vi "Comments.Add Device Description.vi"(8 "error in (no error)":errorcluster, 11 "Control Experiment in":refnum<class "Control Experiment.lvclass">) -> (0 "error out":errorcluster, 3 "Control Experiment out":refnum<class "Control Experiment.lvclass">)   [LabVIEW 2016, in "Control Experiment.lvclass"]
uses:
  Control Experiment.lvclass
  Control Experiment.lvclass/Control Experiment.ctl
panel:
  out "Device Description":string
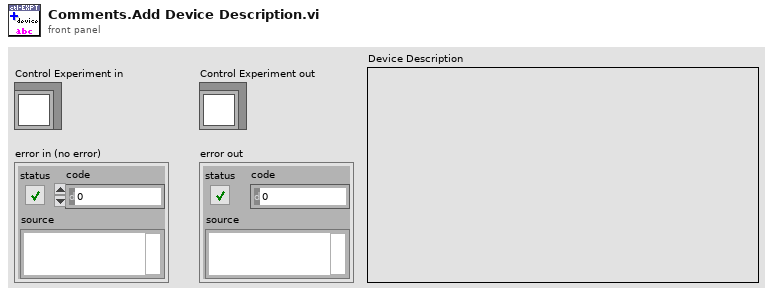
[diagram p1: front panel]
types:
  T1 = typedef "Control Experiment.lvclass/Instrument--enum.ctl" = enum16{"PPMS", "PPMS2", "MFP3D", "CYPHER", "THz1", "THz2", "MNK", "CF900", "JEOL", "AGILENT", "EBL"}
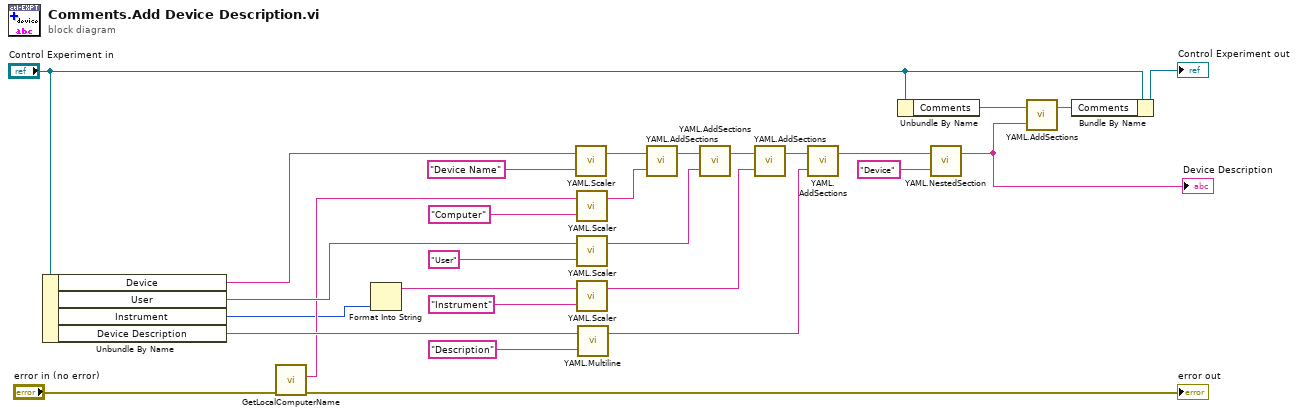
[diagram p0: block diagram]
diagram:
  n1 = Unbundle By Name("Control Experiment in") -> ("Device"=w8:string, "User"=w12:string, "Instrument"=w6:T1, "Device Description"=w17:string)
  n2 = call <userlib>:"GetLocalComputerName.vi"("error in (no error)"="error in (no error)") -> ("error out"=→"error out":errorcluster, "Name"=w10:string)  [unwired: 8 in, 1 out]
  n3 = Format Into String(w6) -> (resulting string=w15:string)  [unwired: 3 in, 1 out]
  n4 = call "YAML.Scaler.vi"("Key"="Device Name" ("string"), "Scaler"=w8) -> ("Output"=w26:string)  [unwired: 1 in]
  n5 = call "YAML.Scaler.vi"("Key"="Computer" ("string"), "Scaler"=w10) -> ("Output"=w18:string)  [unwired: 1 in]
  n6 = call "YAML.Scaler.vi"("Key"="User" ("string"), "Scaler"=w12) -> ("Output"=w20:string)  [unwired: 1 in]
  n7 = call "YAML.Scaler.vi"("Key"="Instrument" ("string"), "Scaler"=w15) -> ("Output"=w21:string)  [unwired: 1 in]
  n8 = call "YAML.Multiline.vi"("Key"="Description" ("string"), "Multiline"=w17) -> ("Output"=w22:string)  [unwired: 1 in]
  n9 = call "YAML.AddSections.vi"("Section 2"=w18, "Section 1"=w26) -> ("Output"=w19:string)  [unwired: 1 in]
  n10 = call "YAML.AddSections.vi"("Section 2"=w20, "Section 1"=w19) -> ("Output"=w23:string)  [unwired: 1 in]
  n11 = call "YAML.AddSections.vi"("Section 2"=w21, "Section 1"=w23) -> ("Output"=w24:string)  [unwired: 1 in]
  n12 = call "YAML.AddSections.vi"("Section 2"=w22, "Section 1"=w24) -> ("Output"=w27:string)  [unwired: 1 in]
  n13 = Unbundle By Name("Control Experiment in") -> ("Comments"=w2:string)
  n14 = call "YAML.NestedSection.vi"("Section Key"="Device" ("string"), "Nested Section"=w27) -> ("String"=w1:string)  [unwired: 1 in]
  "Device Description" <- w1
  n15 = call "YAML.AddSections.vi"("Section 2"=w1, "Section 1"=w2) -> ("Output"=w28:string)  [unwired: 1 in]
  n16 = Bundle By Name(cluster="Control Experiment in", "Comments"=w28) -> (→"Control Experiment out":refnum<class "Control Experiment.lvclass">)
